vi "SaveOneSweep.vi"(5 "Position":T1[](array[typedef]), 7 "SectionProperties":T3, 8 "error in (no error)":errorcluster, 9 ".csv file from N5222A":string, 10 "Temperature, deg C":dbl, 11 "FileMerge in":refnum<class "FileMerge.lvclass">) -> (0 "error out":errorcluster, 3 "FileMerge out":refnum<class "FileMerge.lvclass">)   [LabVIEW 2019, in "FileMerge.lvclass"]
doc: "Read through existing file until\n1. New record matches an old record.\n2. New record enumeration is < the next existing file record enumeration.\n3. Return file contents up to the point of match or <"
uses:
  FileMerge.lvclass
  Datalog/DatalogSubvis/SearchableTag.ctl
  Sequence/SequenceSubvis/RF Direction.ctl
  Sequence/SequenceSubvis/PolarizationSelect.ctl
  APARMainSubvis/VXM Public API/singleAxisMoveDef.ctl
  APARMainSubvis/VXM Public API/mmWaveAxis.ctl
  Datalog/DataLog.lvclass
  ExistingFileMgr/ExistingFileMgr.lvclass
panel:
  out "case":u32(ring) items=["Match"=1, "Insert"=2, "Not Found"=4]
  out "starting File Index":i64 format="%.9p"
  out "Step N of 131,072":i32
  out "Next File Index":i64 format="%.9p"
  out "i":i32
  # "1 match\n2 next record\n4 not found"
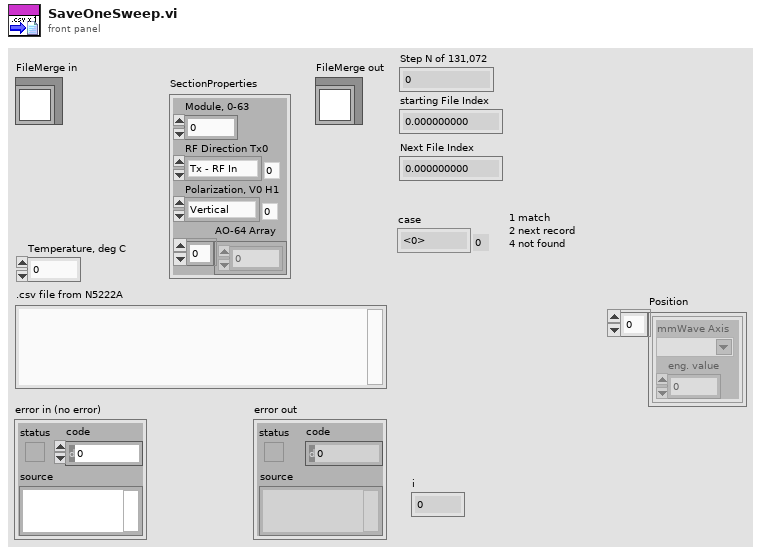
[diagram p1: front panel]
types:
  T1 = typedef "singleAxisMoveDef.ctl" = cluster{"mmWave Axis":T2, "eng. value":dbl}
  T2 = typedef "mmWaveAxis.ctl" = string
  T3 = typedef "DataLog.lvclass/SearchableTag.ctl" = cluster{"Module, 0-63":i32, "RF Direction Tx0":T4, "Polarization, V0 H1":T5, "AO-64 Array":dbl[]}
  T4 = typedef "RF Direction.ctl" = enum16{"Tx - RF In", "Rx - RF Out"}
  T5 = typedef "PolarizationSelect.ctl" = enum16{"Vertical", "Horizontal"}
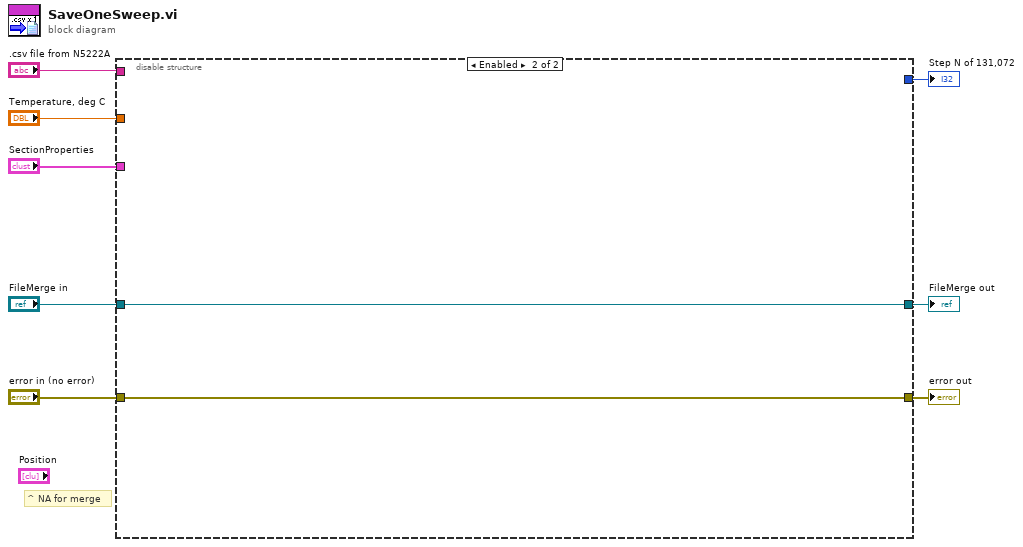
[diagram p0: block diagram]
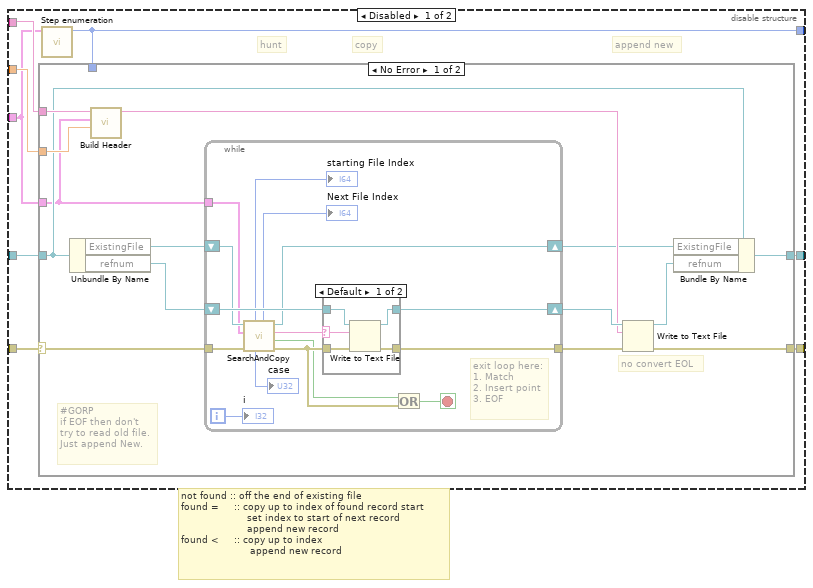
[diagram p2: hidden frame]
diagram:
  # "^ NA for merge"
  n1 = disable-structure shown="Enabled" {
    disable-tunnel: "error in (no error)" -> [w16 w55]
    disable-tunnel: [w15 w55] -> w7
    disable-tunnel: "FileMerge in" -> [w14 w56]
    disable-tunnel: [w13 w56] -> w5
    disable-tunnel: ".csv file from N5222A" -> [w12 _]
    disable-tunnel: "Temperature, deg C" -> [w11 _]
    disable-tunnel: "SectionProperties" -> [w10 _]
    disable-tunnel: [w9 _] -> w1
    frame Disabled {
      # "append new"
      # "copy"
      # "hunt"
      # "not found :: off the end of existing file\nfound =     :: copy up to index of found record start\n                      set index to start of next record\n                      append new record\nfound <     :: copy up to index\n                       append new record"
      n2 = call "Step enumeration.vi"("SweepProperties"=w10) -> ("Step N of 131,072"=w9:i32)  [unwired: 10 in]
      n3 = case shown="No Error" w16 {
        selector: w16 -> [w23 w54]
        tunnel: [w25 w54] -> w15
        tunnel: [w27 w53] -> w13
        tunnel: w14 -> [w28 w53]
        tunnel: w10 -> [w24 _]
        tunnel: w12 -> [w30 _]
        tunnel: w11 -> [w29 _]
        tunnel: w9 -> [_ _]
        frame No Error {
          # "#GORP\nif EOF then don't\ntry to read old file.\nJust append New."
          # "no convert EOL"
          n4 = Unbundle By Name(w28) -> ("ExistingFile"=w20:refnum<class "ExistingFileMgr.lvclass">, "refnum"=w19:refnum<file>)
          n5 = call "Build Header.vi"("Temp, deg C"=w29, "SectionProperties"=w24, "PNA .csv File"=w30) -> ("One Record"=w21:string)  [unwired: 8 in]
          n6 = while {
            tunnel: w24 -> [w41]
            shift-right: [w42] -> w26
            shift-left: w19 -> [w45]
            shift-right: [w43] -> w17
            shift-left: w20 -> [w44]
            tunnel: w23 -> [w38]
            tunnel: [w37] -> w22
            i -> [w39]
            stop <- w34 stop-if-true
            # "exit loop here:\n1. Match\n2. Insert point\n3. EOF"
            n7 = call "SearchAndCopy.vi"("error in (no error)"=w38, "SectionProperties"=w41, "ExistingFileMgr in"=w44) -> ("error out"=w36:errorcluster, "Found index or EOF"=w35:bool, "Existing File Chunk to copy"=w40:string, "ExistingFileMgr out"=w43:refnum<class "ExistingFileMgr.lvclass">, "Next File Index"=→"Next File Index":i64, "case"=→"case":u32, "starting File Index"=→"starting File Index":i64)  [unwired: 2 out]
            n8 = case shown="Default" w40 {
              selector: w40 -> [w46 _]
              tunnel: w45 -> [w50 w52]
              tunnel: [w49 w52] -> w42
              tunnel: [w48 w51] -> w37
              tunnel: w36 -> [w47 w51]
              frame Default {
                n9 = Write to Text File(file (use dialog)=w50, text=w46, error in=w47) -> (refnum out=w49:refnum<file>, error out=w48:errorcluster)  [unwired: 1 in, 1 out]
              }
              frame "" {
              }
            }
            n10 = Or(x=w35, y=w36) -> (x .or. y?=w34:bool)
            "i" <- w39
          }
          n11 = Write to Text File(file (use dialog)=w26, text=w21, error in=w22) -> (refnum out=w18:refnum<file>, error out=w25:errorcluster)  [unwired: 1 in, 1 out]
          n12 = Bundle By Name(cluster=w28, "ExistingFile"=w17, "refnum"=w18) -> (w27:refnum<class "FileMerge.lvclass">)
        }
        frame Error {
        }
      }
    }
    frame Enabled {
    }
  }
  "error out" <- w7
  "FileMerge out" <- w5
  "Step N of 131,072" <- w1
